vi "Handling DI scada.vi"(8 "error in":errorcluster, 10 "DI_reorder_table":i32[](array[numeric]), 11 "OPC UA1.Client refnum":T2) -> (0 "error":errorcluster, 1 "DIALRState":errorcluster[](array[cluster]), 2 "DI_State":T1[](array[typedef]), 3 "DI":bool[](array[boolean]), 4 "connect":bool)   [LabVIEW 2019, in "Inputs.lvlib"]
uses:
  <vilib>/OPCUA/controls/OPC UA Client Refnum.ctl
  <vilib>/OPCUA/controls/NodeIds.ctl
  <vilib>/OPCUA/controls/NodeId.ctl
  <vilib>/OPCUA/client/Multiple Read Int32 Array.vi
  Inputs.lvlib
  <vilib>/OPCUA/NI OPC UA Client.lvlib
  <vilib>/OPCUA/client/Multiple Read Bool Array.vi
  Ctl/Parameter State.ctl
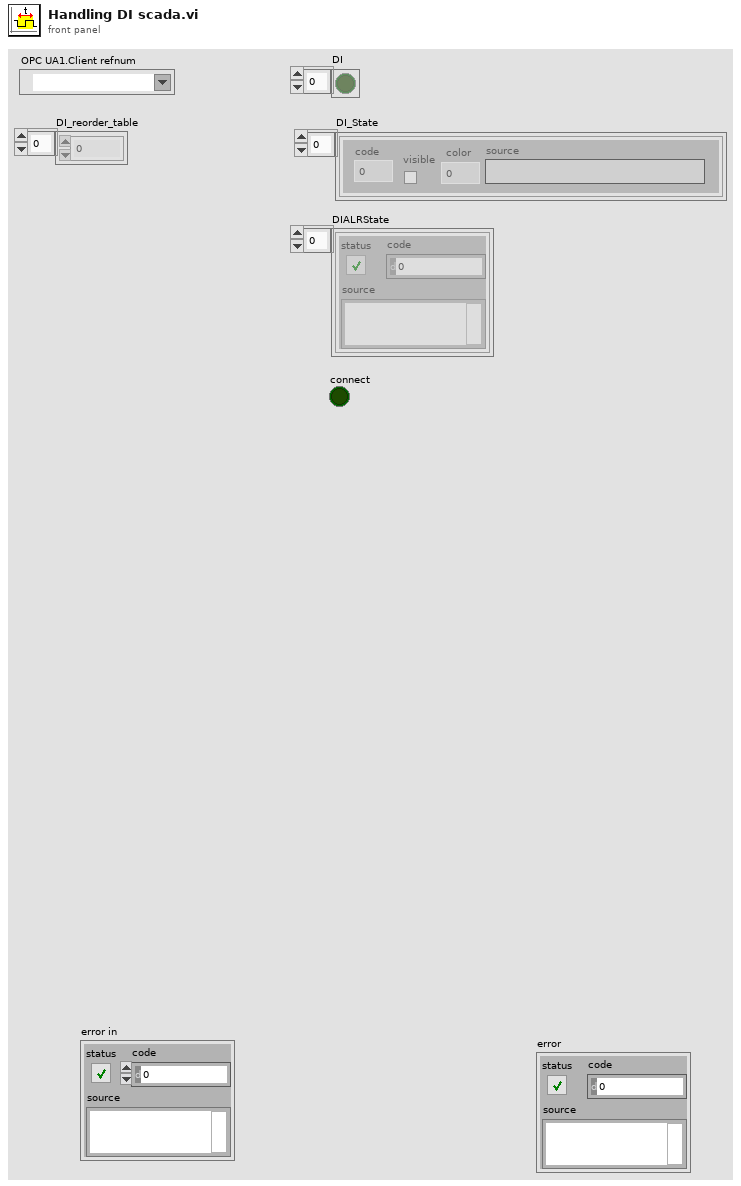
[diagram p1: front panel]
types:
  T1 = typedef "Inputs.lvlib/Parameter State.ctl" = cluster{"code":i32, "visible":bool, "color":u32, "source":string}
  T2 = typedef "OPC UA Client Refnum.ctl" = refnum<k21>
  T3 = typedef "NodeIds.ctl" = T4[]
  T4 = typedef "NodeId.ctl" = string
  T5 = typedef "OPC UA StatusCode.ctl" = u32
  T6 = cluster{"node ID":T4, "values ":bool[], "timestamp":timestamp, "status":T5}[]
  T7 = cluster{"node ID":T4, "values ":i32[], "timestamp":timestamp, "status":T5}[]
  T8 = cluster{"node ID":T4, "values ":bool[], "timestamp":timestamp, "status":T5}
  T9 = cluster{"node ID":T4, "values ":i32[], "timestamp":timestamp, "status":T5}
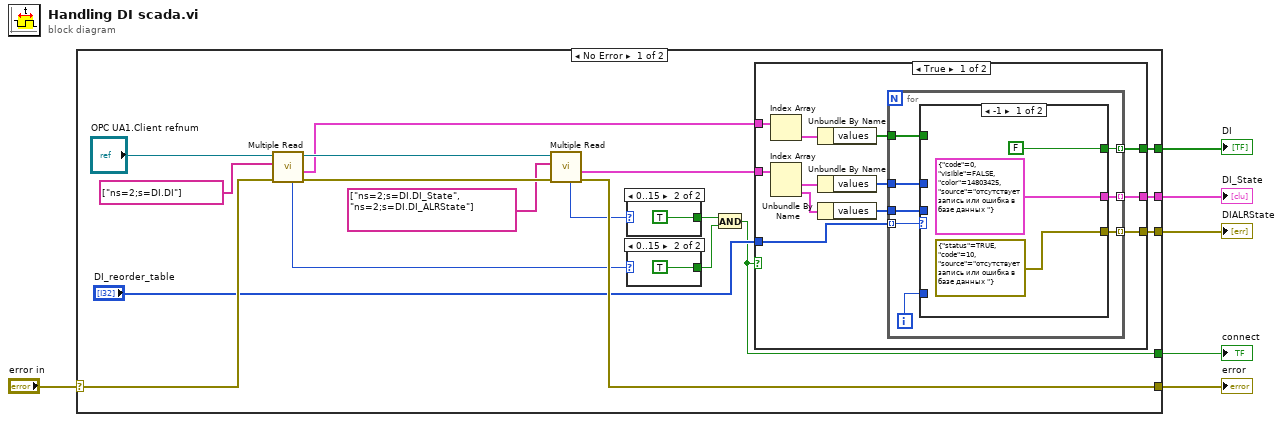
[diagram p0: block diagram]
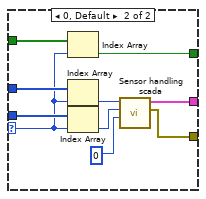
[diagram p2: hidden frame]
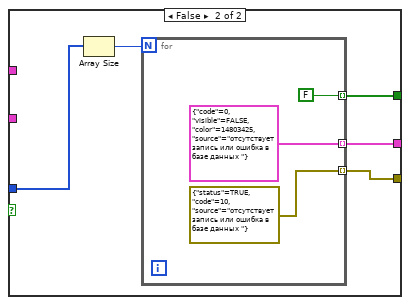
[diagram p3: hidden frame]
diagram:
  n1 = case shown="No Error" "error in" {
    selector: "error in" -> [w24 w68]
    tunnel: [w23 w68] -> w5
    tunnel: [w7 _] -> w4
    tunnel: [w9 _] -> w1
    tunnel: [w10 _] -> w3
    tunnel: [w8 _] -> w2
    frame No Error {
      n2 = call-poly <vilib>:"Multiple Read.vi"("error in (no error)"=w24, "node IDs"=T3 ["ns=2;s=DI.DI"] ("OPC UA.node IDs"), "OPC UA client refnum in"="OPC UA1.Client refnum") -> ("error out"=w20:errorcluster, "results"=w13:T6, "OPC UA client refnum out"=w21:T2, "service status"=w18:T5)  [unwired: 5 in]
      n3 = call-poly <vilib>:"Multiple Read.vi"("error in (no error)"=w20, "node IDs"=T3 ["ns=2;s=DI.DI_State", "ns=2;s=DI.DI_ALRState"] ("OPC UA.node IDs"), "OPC UA client refnum in"=w21) -> ("error out"=w23:errorcluster, "results"=w12:T7, "service status"=w17:T5)  [unwired: 5 in, 1 out]
      n4 = case shown="0..15" w17 {
        tunnel: [_ TRUE] -> w16
        frame 16.., Default {
        }
        frame 0..15 {
        }
      }
      n5 = case shown="0..15" w18 {
        tunnel: [_ TRUE] -> w15
        frame 16.., Default {
        }
        frame 0..15 {
        }
      }
      n6 = And(x=w16, y=w15) -> (x .and. y?=w10:bool)
      n7 = case shown="True" w10 {
        tunnel: w13 -> [w35 _]
        tunnel: w12 -> [w34 _]
        tunnel: "DI_reorder_table" -> [w29 w61]
        tunnel: [w26 w60] -> w9
        tunnel: [w25 w59] -> w8
        tunnel: [w27 w58] -> w7
        frame True {
          n8 = Index Array(array=w35) -> (element=w36:T8)  [unwired: 1 in]
          n9 = Index Array(array=w34) -> (element #1=w33:T9, element #2=w31:T9)  [unwired: 2 in]
          n10 = Unbundle By Name(w36) -> ("values"=w32:bool[])
          n11 = Unbundle By Name(w33) -> ("values"=w30:i32[])
          n12 = Unbundle By Name(w31) -> ("values"=w28:i32[])
          n13 = for {
            tunnel: w32 -> [w44]
            tunnel: w29 -> [w40] mode=indexing
            tunnel: [w43] -> w26 mode=indexing
            tunnel: w28 -> [w42]
            tunnel: [w41] -> w25 mode=indexing
            tunnel: w30 -> [w39]
            tunnel: [w38] -> w27 mode=indexing
            i -> [w37]
            n14 = case shown="-1" w40 {
              selector: w40 -> [_ w50]
              tunnel: w44 -> [_ w57]
              tunnel: [FALSE ("Boolean") w49] -> w43
              tunnel: w42 -> [_ w56]
              tunnel: [T1 {"code"=0, "visible"=FALSE, "color"=14803425, "source"="отсутствует запись или ошибка в базе данных "} ("STATE") w52] -> w41
              tunnel: w39 -> [_ w55]
              tunnel: [errorcluster {"status"=TRUE, "code"=10, "source"="отсутствует запись или ошибка в базе данных "} ("ALRSTATE") w51] -> w38
              tunnel: w37 -> [_ _]
              frame -1 {
              }
              frame 0, Default {
                n15 = Index Array(array=w57, index=w50) -> (element=w49:bool)
                n16 = Index Array(array=w55, index=w50) -> (element=w54:i32)
                n17 = Index Array(array=w56, index=w50) -> (element=w53:i32)
                n18 = call "Sensor handling scada.vi"("color schema"=0, "AI_ALRState"=w53, "AI_State"=w54) -> ("ALRSTATE"=w51:errorcluster, "STATE"=w52:T1)  [unwired: 7 in]
              }
            }
          }
        }
        frame False {
          n19 = Array Size(array=w61) -> (size(s)=w62:i32)
          n20 = for {
            N: w62 -> [_]
            tunnel: [FALSE ("Boolean")] -> w60 mode=indexing
            tunnel: [T1 {"code"=0, "visible"=FALSE, "color"=14803425, "source"="отсутствует запись или ошибка в базе данных "} ("STATE")] -> w59 mode=indexing
            tunnel: [errorcluster {"status"=TRUE, "code"=10, "source"="отсутствует запись или ошибка в базе данных "} ("ALRSTATE")] -> w58 mode=indexing
          }
        }
      }
    }
    frame Error {
    }
  }
  "error" <- w5
  "DIALRState" <- w4
  "connect" <- w3
  "DI" <- w1
  "DI_State" <- w2
